vi "Destroy Client.vi"(8 "error in (no error)":errorcluster, 11 "Client in":refnum<class "Client.lvclass">) -> (0 "error out":errorcluster, 3 "Client out":refnum<class "Client.lvclass">)   [LabVIEW 2013, in "MQTT Server.lvlib" / "Client.lvclass"]
uses:
  Client.lvclass
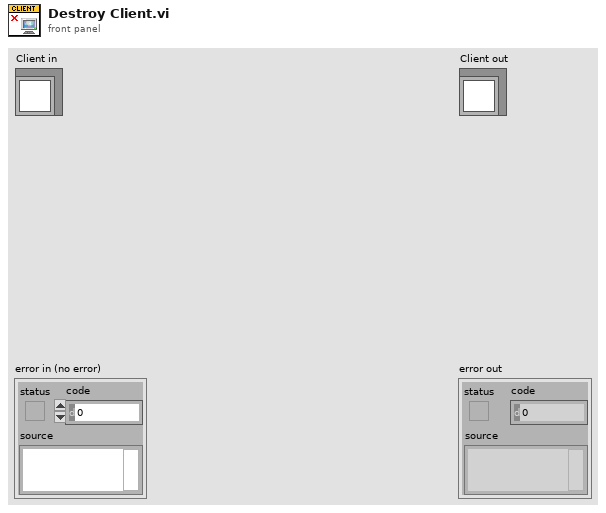
[diagram p1: front panel]
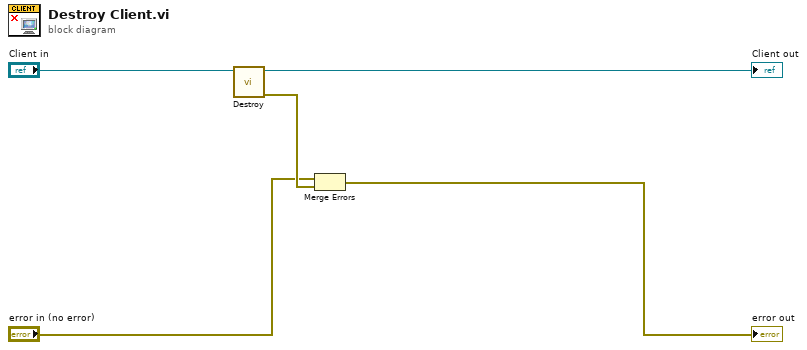
[diagram p0: block diagram]
diagram:
  n1 = call-dynamic "Destroy.vi"("MQTT_Base in"="Client in") -> ("error out"=w3:errorcluster, "MQTT_Base out"=→"Client out":refnum<class "Client.lvclass">)  [unwired: 9 in]
  n2 = Merge Errors("error in (no error)", w3) -> (→"error out":errorcluster)
